vi "Write U32.vi"(8 "error in (no error)":errorcluster, 10 "U32":u32, 11 "Event in":refnum<class "Event U32.lvclass">) -> (0 "error out":errorcluster, 3 "Event out":refnum<class "Event U32.lvclass">)   [LabVIEW 2017, in "Event Actors.lvlib" / "Event U32.lvclass"]
uses:
  Event U32.lvclass
  Event U32.lvclass/Event U32.ctl
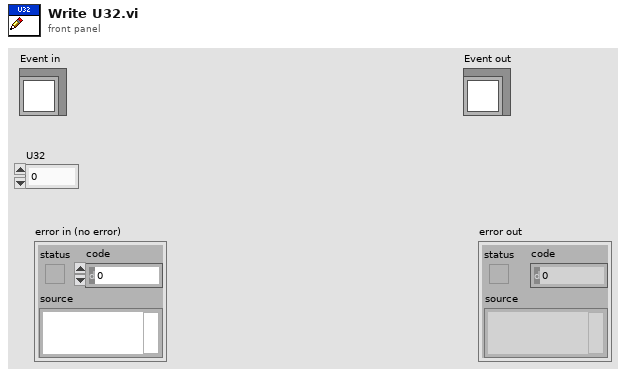
[diagram p1: front panel]
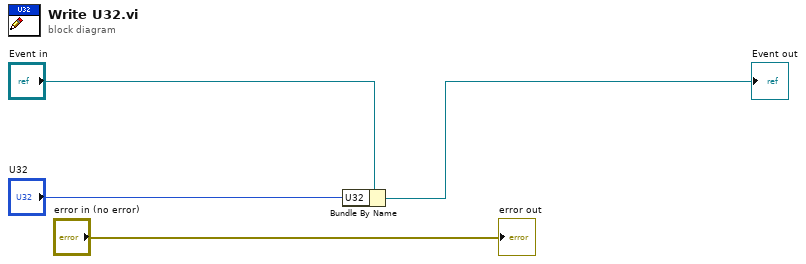
[diagram p0: block diagram]
diagram:
  n1 = Bundle By Name(cluster="Event in", "U32"="U32") -> (→"Event out":refnum<class "Event U32.lvclass">)
  "error out" <- "error in (no error)"
